vi "vertical_bar_inside_brackets.vi"(8 "error in (no error)":errorcluster, 11 "Instrument Command In":string=" :TRIGger:AND:ENABle {{ON | 1} | {OFF | 0}}") -> (0 "error out":errorcluster, 2 "Boolean":bool, 3 "Instrument Command Out":string)   [LabVIEW 2018]
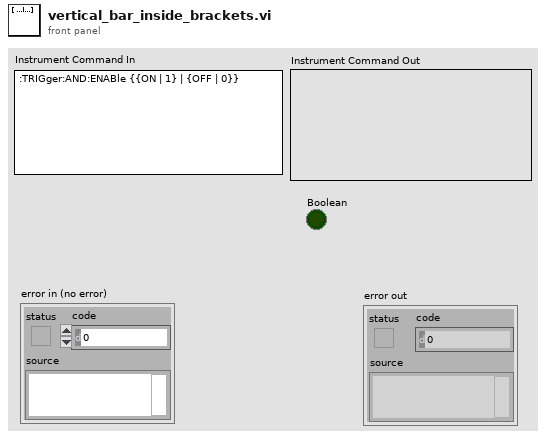
[diagram p1: front panel]
types:
  T1 = cluster{"Start Sting":string, "End String":string}[]
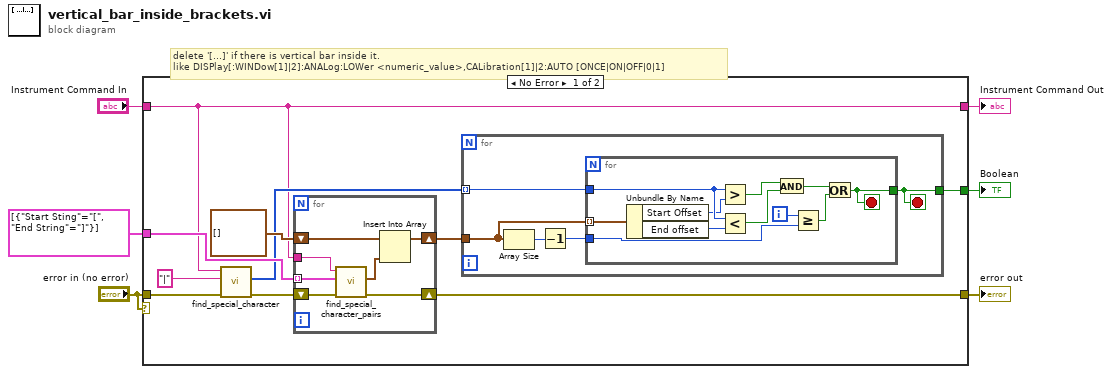
[diagram p0: block diagram]
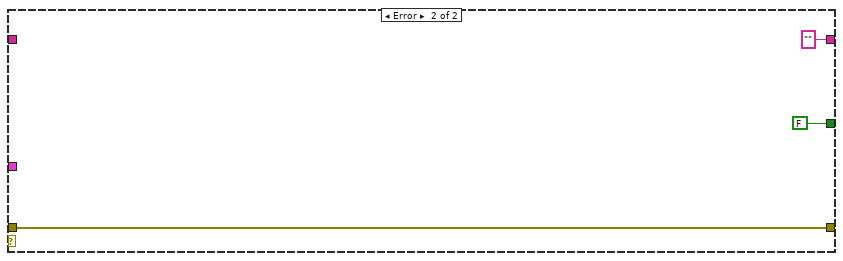
[diagram p2: hidden frame]
diagram:
  # "delete '[...]' if there is vertical bar inside it.\nlike DISPlay[:WINDow[1]|2]:ANALog:LOWer <numeric_value>,CALibration[1]|2:AUTO [ONCE|ON|OFF|0|1]"
  n1 = case shown="No Error" "error in (no error)" {
    tunnel: T1 [{"Start Sting"="[", "End String"="]"}] -> [w15 _]
    tunnel: "Instrument Command In" -> [w7 _]
    tunnel: [w7 "" ("result string")] -> w4
    tunnel: "error in (no error)" -> [w9 w42]
    tunnel: [w10 w42] -> w3
    tunnel: [w8 FALSE] -> w1
    frame No Error {
      n2 = call "find_special_character.vi"("error in (no error)"=w9, "Character"="|" ("Start Character"), "Command String"=w7) -> ("error out"=w11:errorcluster, "Offset Array"=w13:i32[])  [unwired: 7 out]
      n3 = for {
        tunnel: w7 -> [w39]
        tunnel: w15 -> [w38] mode=indexing
        shift-right: [w35] -> w12
        shift-left: cluster{"Start Offset":i32, "End offset":i32}[] [] ("Pair Offset") -> [w36]
        shift-right: [w33] -> w10
        shift-left: w11 -> [w34]
        n4 = call "find_special_character_pairs.vi"("error in (no error)"=w34, "String Pair"=w38, "Command String"=w39) -> ("error out"=w33:errorcluster, "Pair Offset"=w37:cluster{"Start Offset":i32, "End offset":i32}[])  [unwired: 7 out]
        n5 = Insert Into Array(array=w36, new element=w37) -> (w35:cluster{"Start Offset":i32, "End offset":i32}[])  [unwired: 1 in]
      }
      n6 = for {
        tunnel: w13 -> [w21] mode=indexing
        tunnel: w12 -> [w20]
        tunnel: [w17] -> w8
        stop <- w17 stop-if-true
        n7 = Array Size(array=w20) -> (size(s)=w19:i32)
        n8 = Decrement(x=w19) -> (x-1=w18:i32)
        n9 = for {
          tunnel: w21 -> [w29]
          tunnel: w20 -> [w32] mode=indexing
          tunnel: w18 -> [w27]
          tunnel: [w22] -> w17
          i -> [w28]
          stop <- w22 stop-if-true
          n10 = Unbundle By Name(w32) -> ("Start Offset"=w24:i32, "End offset"=w23:i32)
          n11 = Greater?(x=w29, y=w24) -> (0:w31:bool)
          n12 = Less?(x=w29, y=w23) -> (x < y?=w30:bool)
          n13 = And(x=w31, y=w30) -> (x .and. y?=w26:bool)
          n14 = Greater Or Equal?(x=w28, y=w27) -> (x >= y?=w25:bool)
          n15 = Or(x=w26, y=w25) -> (x .or. y?=w22:bool)
        }
      }
    }
    frame Error {
    }
  }
  "Instrument Command Out" <- w4
  "error out" <- w3
  "Boolean" <- w1
